vi "GetPathXY.vi"(11 "PathFileRef In":T2) -> (0 "Reached End":bool, 1 "Y":dbl, 2 "X":dbl, 3 "PathFileRef Out":T1, 4 "current index value":dbl, 5 "World XY":cluster{"X":dbl, "Y":dbl})   [LabVIEW 2014]
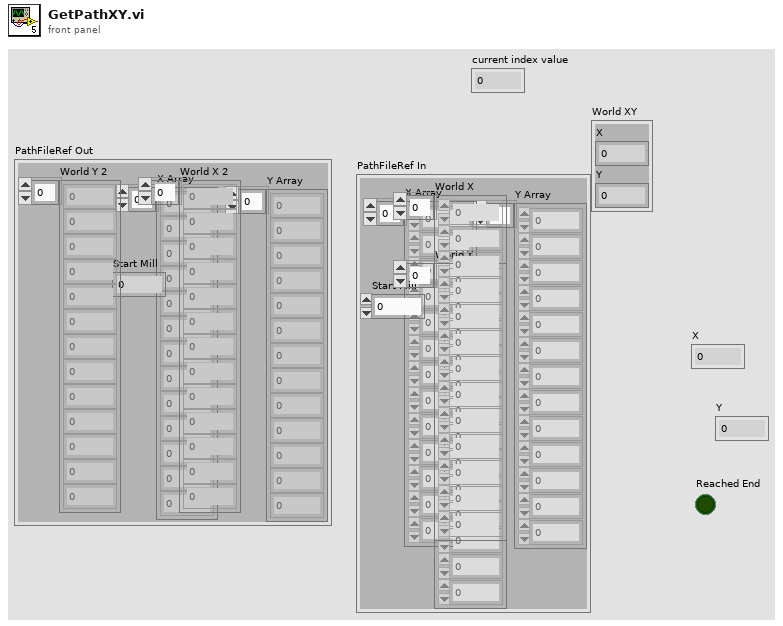
[diagram p1: front panel]
types:
  T1 = cluster{"X Array":dbl[], "Y Array":dbl[], "Start Mill":i32, "World X 2":dbl[], "World Y 2":dbl[]}
  T2 = cluster{"X Array":dbl[], "Y Array":dbl[], "Start Mill":i32, "World Y":dbl[], "World X":dbl[]}
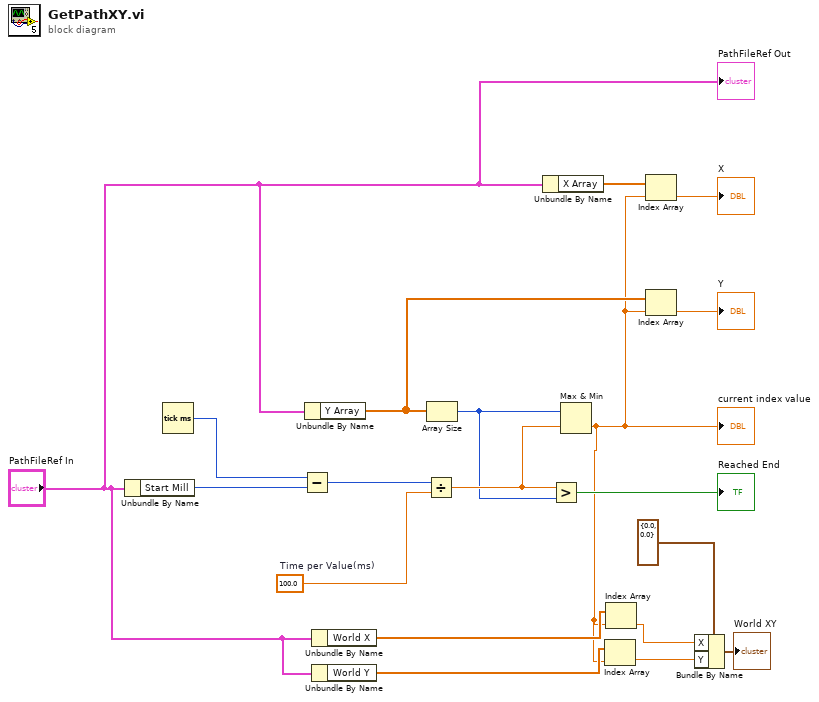
[diagram p0: block diagram]
diagram:
  w16 = 100.0  # Time per Value(ms)
  n1 = Unbundle By Name("PathFileRef In") -> ("Start Mill"=w18:i32)
  n2 = Tick Count (ms)() -> (millisecond timer value=w19:u32)
  n3 = Subtract(x=w19, y=w18) -> (x-y=w17:u32)
  n4 = Unbundle By Name("PathFileRef In") -> ("Y Array"=w12:dbl[])
  n5 = Unbundle By Name("PathFileRef In") -> ("World X"=w8:dbl[])
  n6 = Unbundle By Name("PathFileRef In") -> ("World Y"=w7:dbl[])
  n7 = Divide(x=w17, y=w16) -> (x/y=w15:dbl)
  n8 = Array Size(array=w12) -> (size(s)=w14:i32)
  n9 = Unbundle By Name("PathFileRef In") -> ("X Array"=w10:dbl[])
  n10 = Greater?(x=w15, y=w14) -> (0:→"Reached End":bool)
  n11 = Max & Min(x=w14, y=w15) -> (min(x,y)=w6:dbl)  [unwired: 1 out]
  "current index value" <- w6
  n12 = Index Array(array=w7, index=w6) -> (element=w3:dbl)
  n13 = Index Array(array=w8, index=w6) -> (element=w4:dbl)
  n14 = Index Array(array=w10, index=w6) -> (element=→"X":dbl)
  n15 = Index Array(array=w12, index=w6) -> (element=→"Y":dbl)
  n16 = Bundle By Name(cluster=cluster{"X":dbl, "Y":dbl} {"X"=0.0, "Y"=0.0} ("input cluster"), "X"=w4, "Y"=w3) -> (→"World XY":cluster{"X":dbl, "Y":dbl})
  "PathFileRef Out" <- "PathFileRef In"
